vi "Init.vi"(8 "error in (no error)":errorcluster) -> (0 "error out":errorcluster)   [LabVIEW 2018, in "Template Module.lvlib"]
doc: "Enqueues named action and/or data."
uses:
  Template Module.lvlib
  Private/ctl/Message--enum.ctl
  Private/ctl/State--enum.ctl
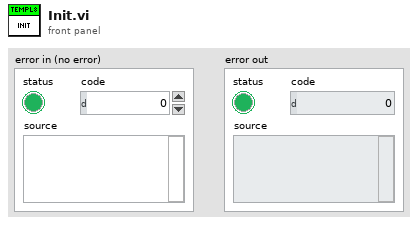
[diagram p1: front panel]
types:
  T1 = typedef "Template Module.lvlib/Message--enum.ctl" = cluster{"State":T2, "Data":variant}
  T2 = typedef "Template Module.lvlib/State--enum.ctl" = enum16{"Init", "Error", "Close"}
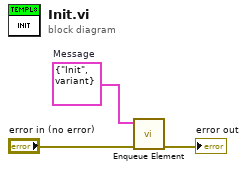
[diagram p0: block diagram]
diagram:
  w1 = T1 {"State"=enum."Init", "Data"=variant}  # Message
  n1 = call "Enqueue Element.vi"("error in"="error in (no error)", "Message"=w1) -> ("error out"=→"error out":errorcluster)  [unwired: 9 in]
